vi "EOL station.vi"(0 "configuration file path":path caption="配置文件的路径", 1 "EOL station msic inf":T1) -> ()   [LabVIEW 2014]
uses:
  Ctl.xio/EOL station msic ctl.ctl
  SubVIS.xio/DataSocket/DataSocket_Tags.ctl
  Ctl.xio/part type.ctl
  <vilib>/Utility/file.llb/Read From Spreadsheet File (string).vi
  SubVIS.xio/DataSocket/Read PLC Vars/Read Bool Var.vi
  SubVIS.xio/DataSocket/Read PLC Vars/Read U32 Var.vi
  SubVIS.xio/DataSocket/Write PLC Vars/Write Bool Var in.vi
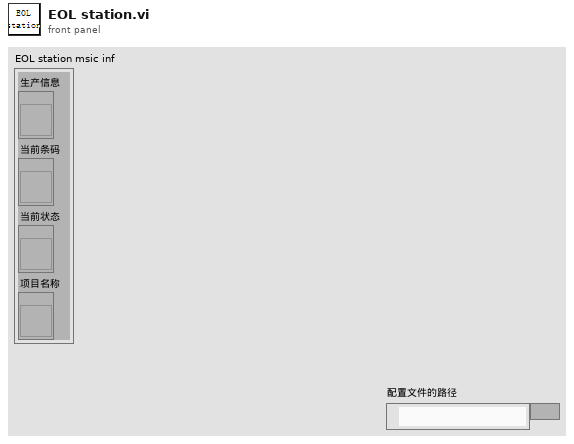
[diagram p1: front panel]
types:
  T1 = cluster{"生产信息":refnum<vi>, "当前条码":refnum<vi>, "当前状态":refnum<vi>, "项目名称":refnum<vi>}
  T2 = typedef "EOL station msic ctl.ctl" = cluster{"configuration file path":path, "DsOut":T3[], "Hopper car information":cluster{"Hopper car code":string, "Hopper car No":string, "plate No":string}, "pallet.produced number":i32, "SQL information":string, "Serial number":i32, "database path":path, "EOL station msic inf":cluster{"生产信息":refnum<vi>, "当前条码":refnum<vi>, "当前状态":refnum<vi>, "项目名称":refnum<vi>}, "part type":T4, "BarCode":string, "scanner resource name out":refnum<visa-resource-name>, "scanner coms":string, "Force value database":string[], "Force value buffer":dbl[], "SN":string, "print inf":string, "2Dcode inf":string, "Pass/Fail":bool}
  T3 = typedef "DataSocket_Tags.ctl" = cluster{"Ds ID":refnum<k13>, "Tag":string}
  T4 = typedef "part type.ctl" = cluster{"项目号":string, "物料代码":string, "零件号":string, "供应商编码":string, "产线编码":string, "客户代码":string, "颜色代码":string, "托盘上限":i32, "加热温度":string, "加热时长":string, "EOL Stations":string}
  T5 = cluster{"Hopper car code":string, "Hopper car No":string, "plate No":string}
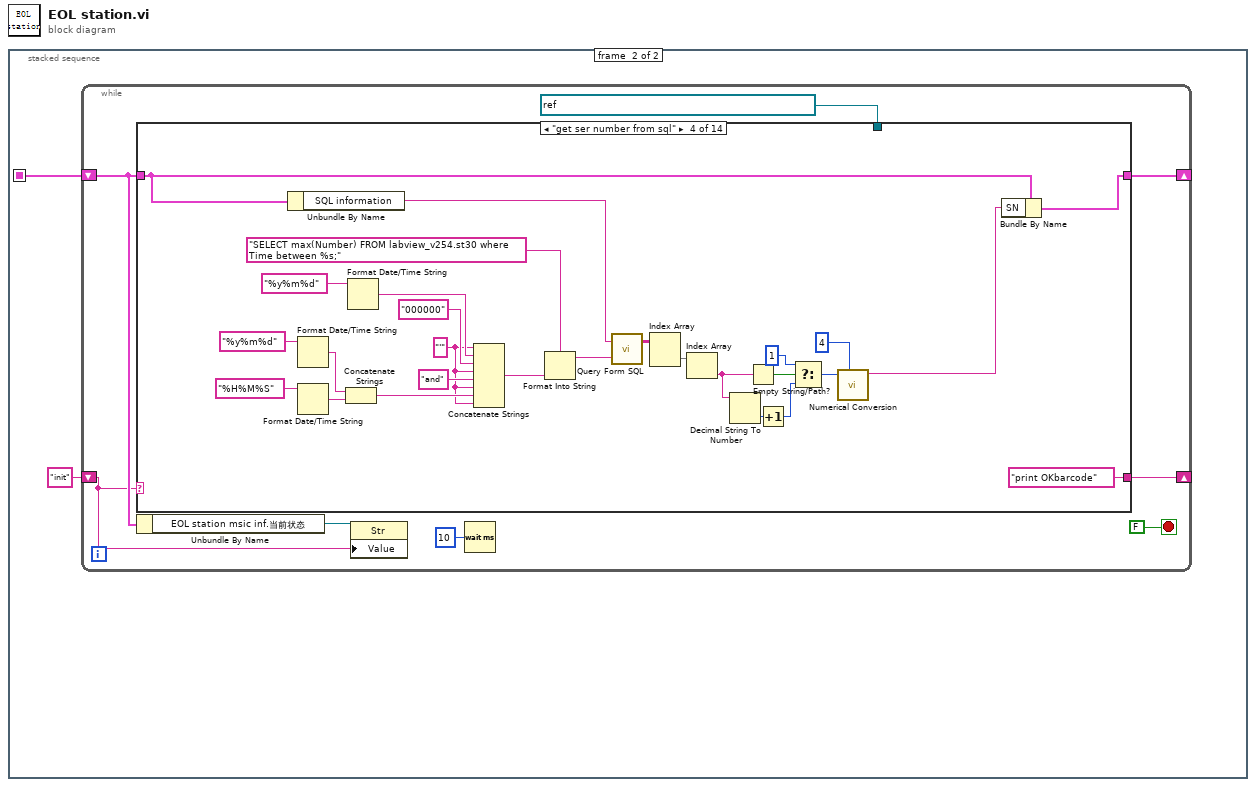
[diagram p0: block diagram]
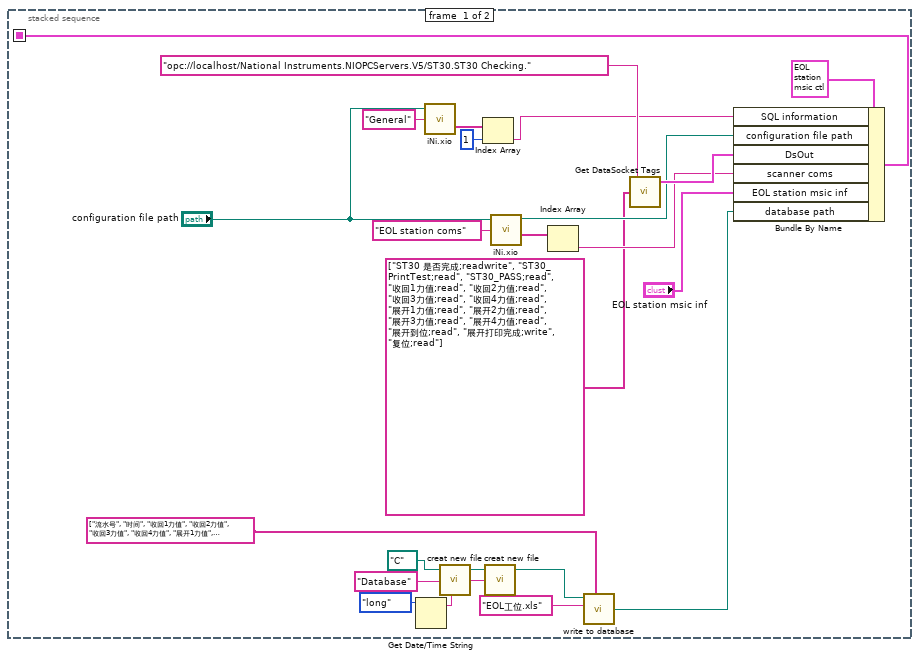
[diagram p2: hidden frame]
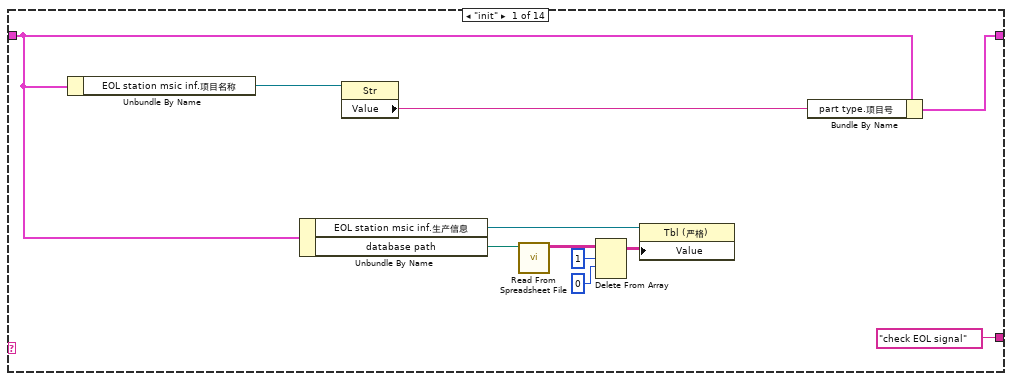
[diagram p3: hidden frame]
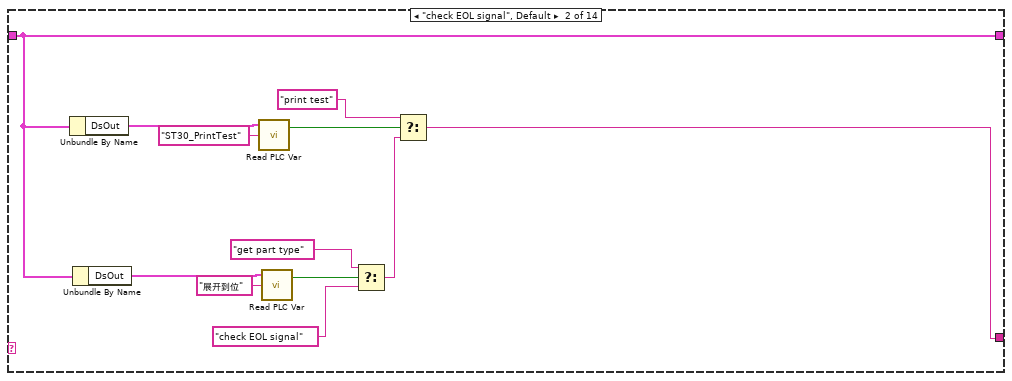
[diagram p4: hidden frame]
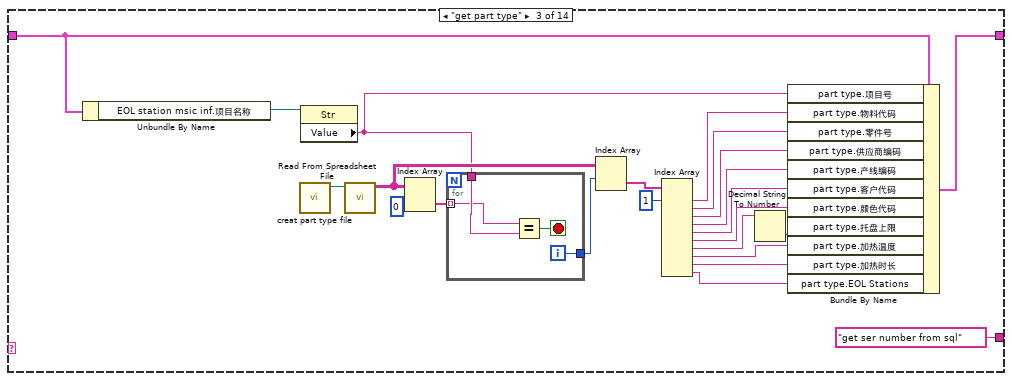
[diagram p5: hidden frame]
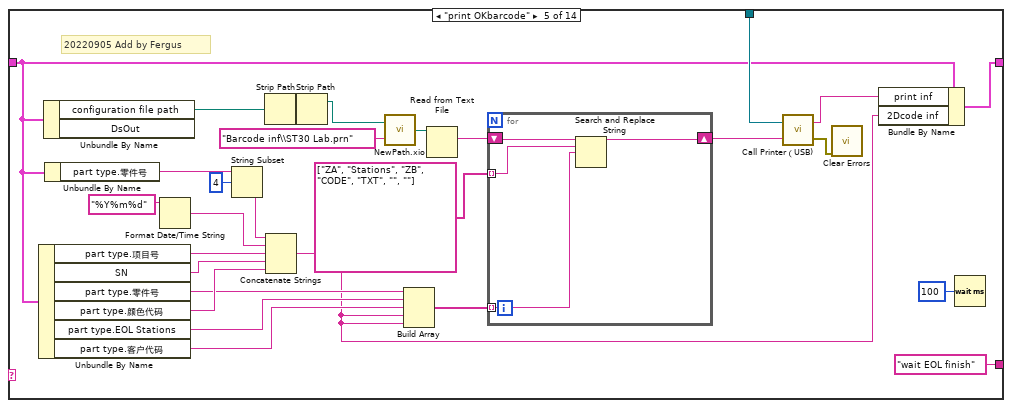
[diagram p6: hidden frame]
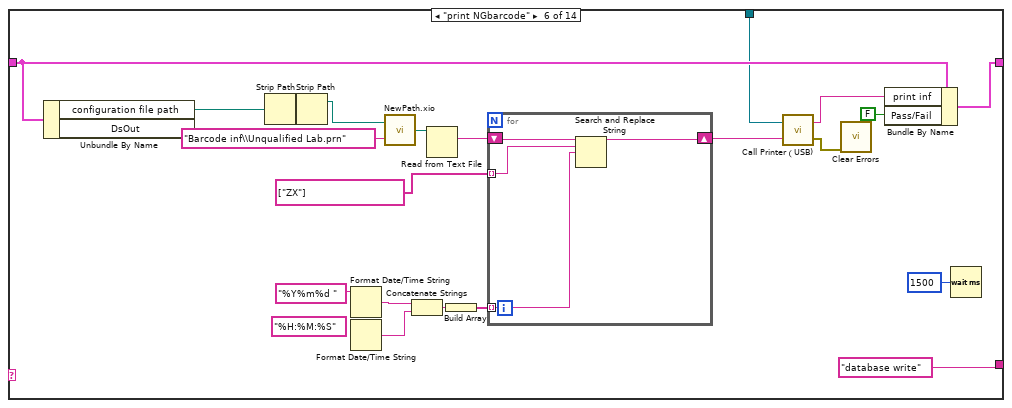
[diagram p7: hidden frame]
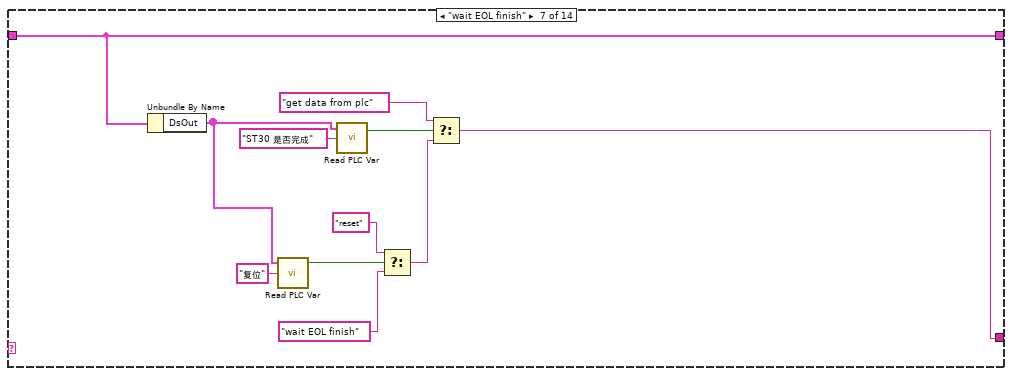
[diagram p8: hidden frame]
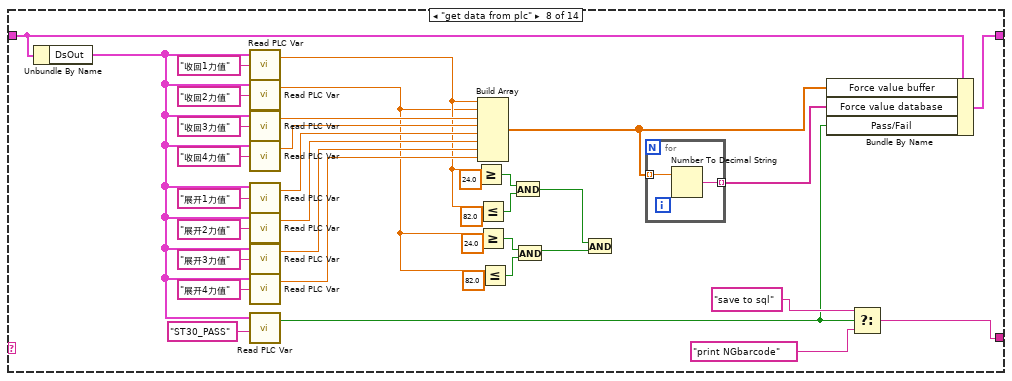
[diagram p9: hidden frame]
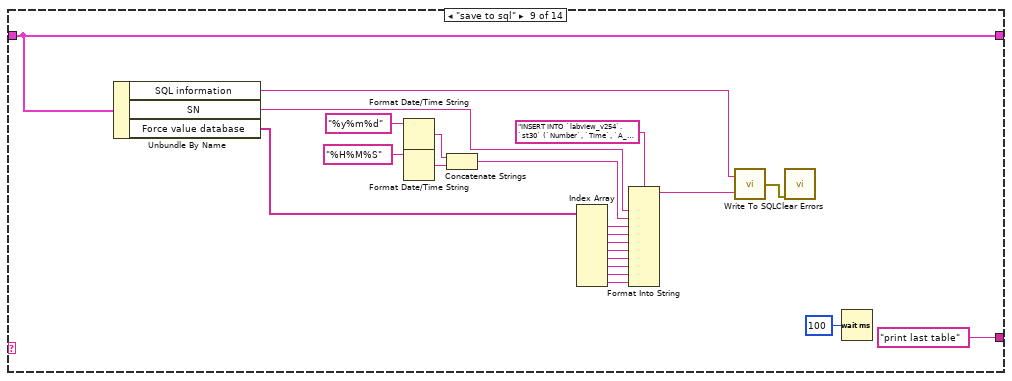
[diagram p10: hidden frame]
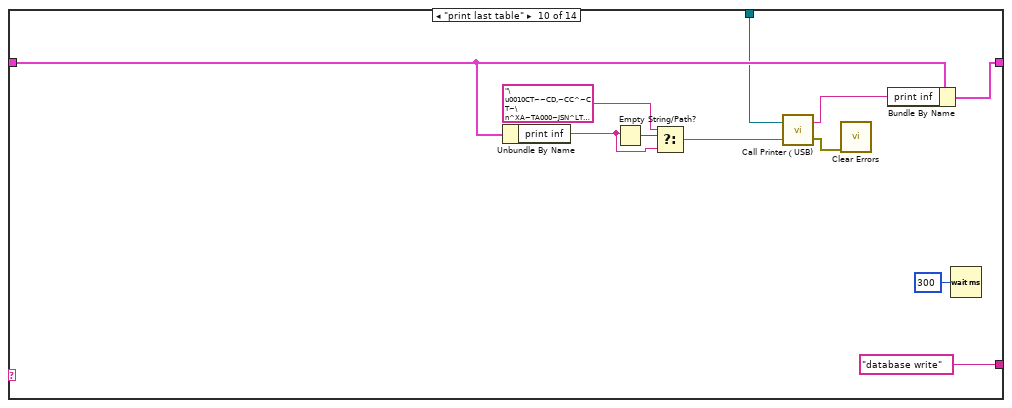
[diagram p11: hidden frame]
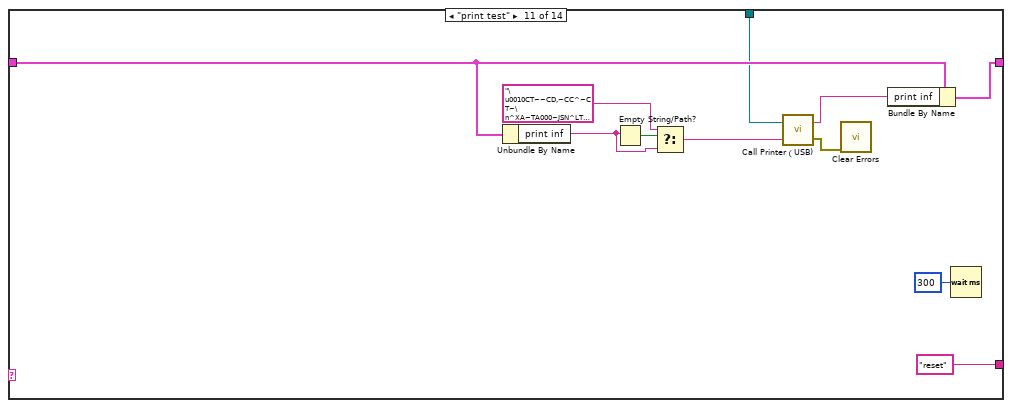
[diagram p12: hidden frame]
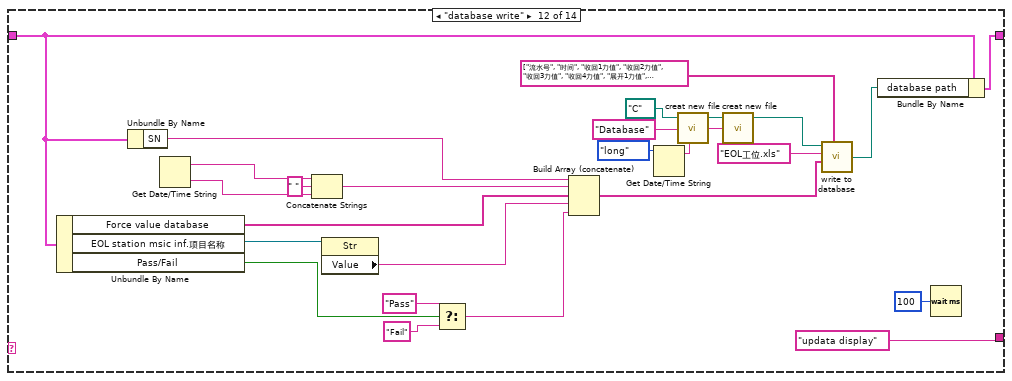
[diagram p13: hidden frame]
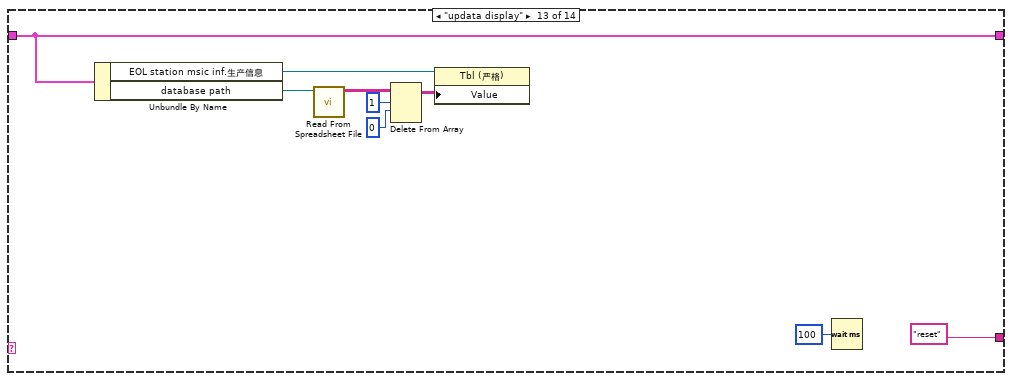
[diagram p14: hidden frame]
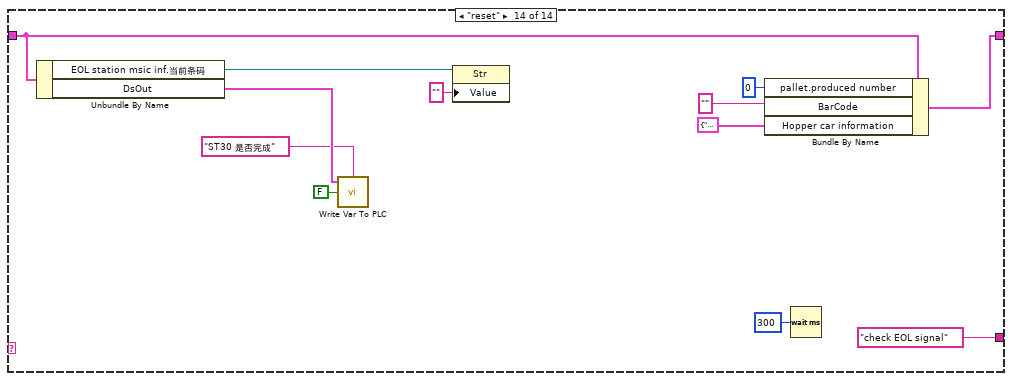
[diagram p15: hidden frame]
diagram:
  n1 = stacked-sequence {
    seq-local: [w17 _] -> [_ w25]
    frame #0 {
      n2 = Get Date/Time String(date format (0)=enum16{"short", "long", "abbreviated"}."long" ("日期格式(0)")) -> (date string=w4:string)  [unwired: 2 in, 1 out]
      n3 = call "iNi.xio.vi"("configuration file path"="configuration file path", "Sections"="General") -> ("Values"=w12:string[])  [unwired: 1 in, 4 out]
      n4 = call "creat new file.vi"("file name"="Database", "path"=path "C:/") -> ("created path"=w6:path)  [unwired: 1 in, 2 out]
      n5 = Index Array(array=w12, index=1 ("索引")) -> (element=w10:string)
      n6 = call "creat new file.vi"("file name"=w4, "path"=w6) -> ("created path"=w5:path)  [unwired: 1 in, 2 out]
      n7 = call "iNi.xio.vi"("configuration file path"="configuration file path", "Sections"="EOL station coms") -> ("configuration file path"=w23:path, "Values"=w21:string[])  [unwired: 1 in, 3 out]
      n8 = Index Array(array=w21) -> (element=w20:string)  [unwired: 1 in]
      n9 = call "write to database.vi"("Header"=string[] ["流水号", "时间", "收回1力值", "收回2力值", "收回3力值", "收回4力值", "展开1力值", "展开2力值", "展开3力值", "展开4力值", "项目号", "Pass/Fail"], "file name"="EOL工位.xls", "path"=w5) -> ("new file path (Not A Path if cancelled)"=w2:path)  [unwired: 3 in]
      n10 = call "Get DataSocket Tags.vi"("All Tags"=string[] ["ST30 是否完成;readwrite", "ST30_PrintTest;read", "ST30_PASS;read", "收回1力值;read", "收回2力值;read", "收回3力值;read", "收回4力值;read", "展开1力值;read", "展开2力值;read", "展开3力值;read", "展开4力值;read", "展开到位;read", "展开打印完成;write", "复位;read"], "URL"="opc://localhost/National Instruments.NIOPCServers.V5/ST30.ST30 Checking.") -> ("DsOut"=w24:T3[])  [unwired: 3 in]
      n11 = Bundle By Name(cluster=T2 {"configuration file path"=path "", "DsOut"=[], "Hopper car information"={"Hopper car code"="", "Hopper car No"="", "plate No"=""}, "pallet.produced number"=0, "SQL information"="", "Serial number"=0, "database path"=path "", "EOL station msic inf"={"生产信息"=refnum, "当前条码"=refnum, "当前状态"=refnum, "项目名称"=refnum}, "part type"={"项目号"="", "物料代码"="", "零件号"="", "供应商编码"="", "产线编码"="", "客户代码"="", "颜色代码"="", "托盘上限"=0, "加热温度"="", "加热时长"="", "EOL Stations"=""}, "BarCode"="", "scanner resource name out"="", "scanner coms"="", "Force value database"=[], "Force value buffer"=[], "SN"="", "print inf"="", "2Dcode inf"="", "Pass/Fail"=FALSE} ("PDF Welding msic ctl"), "SQL information"=w10, "configuration file path"=w23, "DsOut"=w24, "scanner coms"=w20, "EOL station msic inf"="EOL station msic inf", "database path"=w2) -> (w17:T2)
    }
    frame #1 {
      n12 = while {
        shift-right: [w34] -> _
        shift-left: w25 -> [w29]
        shift-right: [w33] -> _
        shift-left: "init" ("event") -> [w28]
        stop <- FALSE stop-if-true
        n13 = case shown="\"get ser number from sql\"" w28 {
          tunnel: w29 -> [w35 w50 w79 w87 w115 w155 w176 w207 w220 w246 w257 w270 w294 w303]
          tunnel: [w45 w50 w58 w90 w120 w153 w176 w206 w220 w249 w260 w283 w294 w307] -> w34
          tunnel: ["check EOL signal" w46 "get ser number from sql" ("f") "print OKbarcode" ("f") "wait EOL finish" ("f") "database write" ("f") w175 w198 "print last table" ("f") "database write" ("f") "reset" ("f") "updata display" ("f") "reset" ("f") "check EOL signal" ("f")] -> w33
          tunnel: refnum<visa-resource-name> "USB0::0x0A5F::0x0081::29J194401307::RAW" ("VISA资源名称") -> [_ _ _ _ w116 w144 _ _ _ w240 w251 _ _ _]
          frame "init" {
            n14 = Unbundle By Name(w35) -> ("EOL station msic inf.项目名称"=w44:refnum<vi>)
            n15 = Unbundle By Name(w35) -> ("EOL station msic inf.生产信息"=w41:refnum<vi>, "database path"=w40:path)
            n16 = property class="Str"(reference=w44) -> ("Value"=w43:string)  [unwired: 1 in, 2 out]
            n17 = call-poly <vilib>:"Read From Spreadsheet File.vi"("file path (dialog if empty)"=w40) -> ("all rows"=w39:string[][])  [unwired: 6 in, 4 out]
            n18 = Delete From Array(array=w39, length=1 ("长度"), index (row)=0 ("索引 (行)")) -> (array with subset deleted=w36:string[][])  [unwired: 1 in, 1 out]
            n19 = property class="Tbl (严格)"(reference=w41, "Value"=w36) -> ()  [unwired: 1 in, 2 out]
            n20 = Bundle By Name(cluster=w35, "part type.项目号"=w43) -> (w45:T2)
          }
          frame "check EOL signal", Default {
            n21 = Unbundle By Name(w50) -> ("DsOut"=w51:T3[])
            n22 = Unbundle By Name(w50) -> ("DsOut"=w57:T3[])
            n23 = call-poly "Read PLC Var.vi"("Tag IN"="ST30_PrintTest", "Ds PLCTags IN"=w51) -> ("Bool Var out"=w49:bool)  [unwired: 1 in, 1 out]
            n24 = call-poly "Read PLC Var.vi"("Tag IN"="展开到位", "Ds PLCTags IN"=w57) -> ("Bool Var out"=w55:bool)  [unwired: 1 in, 1 out]
            n25 = Select(t="get part type" ("f"), s=w55, f="check EOL signal") -> (s? t:f=w48:string)
            n26 = Select(t="print test" ("f"), s=w49, f=w48) -> (s? t:f=w46:string)
          }
          frame "get part type" {
            n27 = Unbundle By Name(w79) -> ("EOL station msic inf.项目名称"=w80:refnum<vi>)
            n28 = call "creat part type file.vi"() -> ("new file path (Not A Path if cancelled)"=w73:path)  [unwired: 11 in]
            n29 = property class="Str"(reference=w80) -> ("Value"=w72:string)  [unwired: 1 in, 2 out]
            n30 = call-poly <vilib>:"Read From Spreadsheet File.vi"("file path (dialog if empty)"=w73) -> ("all rows"=w76:string[][])  [unwired: 6 in, 4 out]
            n31 = Index Array(array=w76, index (col)=0 ("禁用的索引 (列)")) -> (element=w77:string[])  [unwired: 1 in]
            n32 = for {
              tunnel: w77 -> [w81] mode=indexing
              tunnel: [w83] -> w75
              tunnel: w72 -> [w82]
              i -> [w83]
              stop <- w84 stop-if-true
              n33 = Equal?(x=w81, y=w82) -> (x = y?=w84:bool)
            }
            n34 = Index Array(array=w76, index (row)=w75) -> (element=w74:string[])  [unwired: 1 in]
            n35 = Index Array(array=w74, index #1=1 ("索引")) -> (element #1=w69:string, element #2=w68:string, element #3=w67:string, element #4=w66:string, element #5=w64:string, element #6=w65:string, element #7=w62:string, element #8=w61:string, element #9=w60:string, element #10=w59:string)  [unwired: 9 in]
            n36 = Decimal String To Number(string=w62) -> (number=w63:i32)  [unwired: 2 in, 1 out]
            n37 = Bundle By Name(cluster=w79, "part type.项目号"=w72, "part type.物料代码"=w69, "part type.零件号"=w68, "part type.供应商编码"=w67, "part type.产线编码"=w66, "part type.客户代码"=w64, "part type.颜色代码"=w65, "part type.托盘上限"=w63, "part type.加热温度"=w61, "part type.加热时长"=w60, "part type.EOL Stations"=w59) -> (w58:T2)
          }
          frame "get ser number from sql" {
            w101 = "'" ("字符串")
            n38 = Unbundle By Name(w87) -> ("SQL information"=w86:string)
            n39 = Format Date/Time String(time format string (%c)="%y%m%d" ("时间格式字符串(%c)")) -> (date/time string=w104:string)  [unwired: 2 in]
            n40 = Format Date/Time String(time format string (%c)="%H%M%S" ("时间格式字符串(%c)")) -> (date/time string=w105:string)  [unwired: 2 in]
            n41 = Concatenate Strings(w104, w105) -> (w102:string)
            n42 = Format Date/Time String(time format string (%c)="%y%m%d" ("时间格式字符串(%c)")) -> (date/time string=w108:string)  [unwired: 2 in]
            n43 = Concatenate Strings(w101, w108, "000000" ("字符串"), w101, "and" ("字符串"), w101, w102, w101) -> (w100:string)
            n44 = Format Into String(format string="SELECT max(Number) FROM labview_v254.st30 where Time between %s;" ("SQL query"), w100) -> (resulting string=w99:string)  [unwired: 2 in, 1 out]
            n45 = call "Query Form SQL.vi"("SQL query"=w99, "SQL ID"=w86) -> ("data"=w98:string[][])  [unwired: 1 out]
            n46 = Index Array(array=w98) -> (element=w97:string[])  [unwired: 2 in]
            n47 = Index Array(array=w97) -> (element=w93:string)  [unwired: 1 in]
            n48 = Decimal String To Number(string=w93) -> (number=w92:i32)  [unwired: 2 in, 1 out]
            n49 = Empty String/Path?(string/path=w93) -> (empty?=w96:bool)
            n50 = Increment(x=w92) -> (x+1=w91:i32)
            n51 = Select(t=1, s=w96, f=w91) -> (s? t:f=w94:i32)
            n52 = call "Numerical Conversion.vi"("width"=4, "num"=w94) -> ("字符串"=w89:string)  [unwired: 9 in]
            n53 = Bundle By Name(cluster=w87, "SN"=w89) -> (w90:T2)
          }
          frame "print OKbarcode" {
            # "20220905 Add by Fergus"
            n54 = Unbundle By Name(w115) -> ("part type.项目号"=w129:string, "SN"=w123:string, "part type.零件号"=w127:string, "part type.颜色代码"=w128:string, "part type.EOL Stations"=w126:string, "part type.客户代码"=w125:string)
            n55 = Unbundle By Name(w115) -> ("configuration file path"=w138:path)  [unwired: 1 out]
            n56 = Unbundle By Name(w115) -> ("part type.零件号"=w114:string)
            n57 = Format Date/Time String(time format string (%c)="%Y%m%d" ("时间格式字符串(%c)")) -> (date/time string=w130:string)  [unwired: 2 in]
            n58 = String Subset(string=w114, offset (0)=4 ("偏移量(0)")) -> (substring=w112:string)  [unwired: 1 in]
            n59 = Strip Path(path=w138) -> (stripped path=w137:path)  [unwired: 1 out]
            n60 = Concatenate Strings(w112, w130, w129, w123, w128) -> (w119:string)
            n61 = Strip Path(path=w137) -> (stripped path=w136:path)  [unwired: 1 out]
            n62 = call "NewPath.xio.vi"("Append path"="Barcode inf\\ST30 Lab.prn", "Basic path"=w136) -> ("New path"=w134:path)
            n63 = Build Array(w127, w126, w125, w119, w119) -> (w124:string[])
            n64 = Read from Text File(file (use dialog)=w134) -> (text=w133:string)  [unwired: 3 in, 3 out]
            n65 = for {
              shift-right: [w140] -> w122
              shift-left: w133 -> [w143]
              tunnel: string[] ["ZA", "Stations", "ZB", "CODE", "TXT", "", ""] -> [w142] mode=indexing
              tunnel: w124 -> [w141] mode=indexing
              n66 = Search and Replace String(input string=w143, search string=w142, replace string=w141) -> (result string=w140:string)  [unwired: 5 in, 3 out]
            }
            n67 = call "Call Printer（USB).vi"("写入缓冲区"=w122, "VISA资源名称"=w116) -> ("error out"=w118:errorcluster, "Last P"=w121:string)
            n68 = call <vilib>:"Clear Errors.vi"("error in (no error)"=w118) -> ()  [unwired: 5 in, 2 out]
            n69 = Bundle By Name(cluster=w115, "print inf"=w121, "2Dcode inf"=w119) -> (w120:T2)
            n70 = Wait (ms)(milliseconds to wait=u32 100 ("等待时间（毫秒）")) -> ()  [unwired: 1 out]
          }
          frame "print NGbarcode" {
            (unwired) "%H:%M:%S" ("时间格式字符串(%c)")
            n71 = Unbundle By Name(w155) -> ("configuration file path"=w164:path)  [unwired: 1 out]
            n72 = Strip Path(path=w164) -> (stripped path=w163:path)  [unwired: 1 out]
            n73 = Strip Path(path=w163) -> (stripped path=w162:path)  [unwired: 1 out]
            n74 = Format Date/Time String(time format string (%c)="%Y%m%d " ("时间格式字符串(%c)")) -> (date/time string=w151:string)  [unwired: 2 in]
            n75 = Format Date/Time String() -> (date/time string=w150:string)  [unwired: 3 in]
            n76 = call "NewPath.xio.vi"("Append path"="Barcode inf\\Unqualified Lab.prn", "Basic path"=w162) -> ("New path"=w160:path)
            n77 = Concatenate Strings(w151, w150) -> (w149:string)
            n78 = Read from Text File(file (use dialog)=w160) -> (text=w159:string)  [unwired: 3 in, 3 out]
            n79 = Build Array(w149) -> (w157:string[])
            n80 = for {
              shift-right: [w165] -> w156
              shift-left: w159 -> [w168]
              tunnel: string[] ["ZX"] -> [w167] mode=indexing
              tunnel: w157 -> [w166] mode=indexing
              n81 = Search and Replace String(input string=w168, search string=w167, replace string=w166) -> (result string=w165:string)  [unwired: 5 in, 3 out]
            }
            n82 = call "Call Printer（USB).vi"("写入缓冲区"=w156, "VISA资源名称"=w144) -> ("error out"=w148:errorcluster, "Last P"=w154:string)
            n83 = call <vilib>:"Clear Errors.vi"("error in (no error)"=w148) -> ()  [unwired: 5 in, 2 out]
            n84 = Bundle By Name(cluster=w155, "print inf"=w154, "Pass/Fail"=FALSE) -> (w153:T2)
            n85 = Wait (ms)(milliseconds to wait=u32 1500 ("等待时间（毫秒）")) -> ()  [unwired: 1 out]
          }
          frame "wait EOL finish" {
            n86 = Unbundle By Name(w176) -> ("DsOut"=w173:T3[])
            n87 = call-poly "Read PLC Var.vi"("Tag IN"="复位", "Ds PLCTags IN"=w173) -> ("Bool Var out"=w172:bool)  [unwired: 1 in, 1 out]
            n88 = call-poly "Read PLC Var.vi"("Tag IN"="ST30 是否完成", "Ds PLCTags IN"=w173) -> ("Bool Var out"=w178:bool)  [unwired: 1 in, 1 out]
            n89 = Select(t="reset" ("f"), s=w172, f="wait EOL finish") -> (s? t:f=w169:string)
            n90 = Select(t="get data from plc" ("f"), s=w178, f=w169) -> (s? t:f=w175:string)
          }
          frame "get data from plc" {
            n91 = Unbundle By Name(w207) -> ("DsOut"=w183:T3[])
            n92 = call-poly "Read PLC Var.vi"("Tag IN"="收回1力值", "Ds PLCTags IN"=w183) -> ("U32 Var out"=w194:dbl)  [unwired: 1 in, 1 out]
            n93 = call-poly "Read PLC Var.vi"("Tag IN"="收回2力值", "Ds PLCTags IN"=w183) -> ("U32 Var out"=w186:dbl)  [unwired: 1 in, 1 out]
            n94 = call-poly "Read PLC Var.vi"("Tag IN"="收回3力值", "Ds PLCTags IN"=w183) -> ("U32 Var out"=w205:dbl)  [unwired: 1 in, 1 out]
            n95 = call-poly "Read PLC Var.vi"("Tag IN"="收回4力值", "Ds PLCTags IN"=w183) -> ("U32 Var out"=w204:dbl)  [unwired: 1 in, 1 out]
            n96 = call-poly "Read PLC Var.vi"("Tag IN"="展开1力值", "Ds PLCTags IN"=w183) -> ("U32 Var out"=w200:dbl)  [unwired: 1 in, 1 out]
            n97 = call-poly "Read PLC Var.vi"("Tag IN"="展开2力值", "Ds PLCTags IN"=w183) -> ("U32 Var out"=w203:dbl)  [unwired: 1 in, 1 out]
            n98 = call-poly "Read PLC Var.vi"("Tag IN"="展开3力值", "Ds PLCTags IN"=w183) -> ("U32 Var out"=w202:dbl)  [unwired: 1 in, 1 out]
            n99 = call-poly "Read PLC Var.vi"("Tag IN"="展开4力值", "Ds PLCTags IN"=w183) -> ("U32 Var out"=w201:dbl)  [unwired: 1 in, 1 out]
            n100 = call-poly "Read PLC Var.vi"("Tag IN"="ST30_PASS", "Ds PLCTags IN"=w183) -> ("Bool Var out"=w180:bool)  [unwired: 1 in, 1 out]
            n101 = Greater Or Equal?(x=w194, y=24.0) -> (x >= y?=w191:bool)
            n102 = Build Array(w194, w186, w205, w204, w200, w203, w202, w201) -> (w197:dbl[])
            n103 = Less Or Equal?(x=w194, y=82.0) -> (x <= y?=w192:bool)
            n104 = Greater Or Equal?(x=w186, y=24.0) -> (x >= y?=w190:bool)
            n105 = Less Or Equal?(x=w186, y=82.0) -> (x <= y?=w189:bool)
            n106 = And(x=w191, y=w192) -> (x .and. y?=w184:bool)
            n107 = And(x=w190, y=w189) -> (x .and. y?=w185:bool)
            n108 = And(x=w184, y=w185) -> ()  [unwired: 1 out]
            n109 = for {
              tunnel: w197 -> [w217] mode=indexing
              tunnel: [w216] -> w196 mode=indexing
              n110 = Number To Decimal String(number=w217) -> (decimal integer string=w216:string)  [unwired: 1 in]
            }
            n111 = Bundle By Name(cluster=w207, "Force value buffer"=w197, "Force value database"=w196, "Pass/Fail"=w180) -> (w206:T2)
            n112 = Select(t="save to sql" ("f"), s=w180, f="print NGbarcode") -> (s? t:f=w198:string)
          }
          frame "save to sql" {
            n113 = Unbundle By Name(w220) -> ("SQL information"=w222:string, "SN"=w234:string, "Force value database"=w233:string[])
            n114 = Format Date/Time String(time format string (%c)="%y%m%d" ("时间格式字符串(%c)")) -> (date/time string=w237:string)  [unwired: 2 in]
            n115 = Format Date/Time String(time format string (%c)="%H%M%S" ("时间格式字符串(%c)")) -> (date/time string=w238:string)  [unwired: 2 in]
            n116 = Concatenate Strings(w237, w238) -> (w235:string)
            n117 = Index Array(array=w233) -> (element #1=w232:string, element #2=w231:string, element #3=w230:string, element #4=w229:string, element #5=w228:string, element #6=w227:string, element #7=w226:string, element #8=w225:string)  [unwired: 8 in]
            n118 = Format Into String(format string="INSERT INTO `labview_v254`.`st30` (`Number`, `Time`, `A_Data1`, `A_Data2`, `A_Data3`, `A_Data4`, `B_Data1`, `B_Data2`, `B_Data3`, `B_Data4`) VALUES ('%s', '%s', '%s', '%s', '%s', '%s', '%s', '%s', '%s', '%s');" ("初始字符串"), w234, w235, w232, w231, w230, w229, w228, w227, w226, w225) -> (resulting string=w223:string)  [unwired: 2 in, 1 out]
            n119 = call "Write To SQL.vi"("SQL query"=w223, "connection information"=w222) -> ("error out"=w221:errorcluster)
            n120 = call <vilib>:"Clear Errors.vi"("error in (no error)"=w221) -> ()  [unwired: 5 in, 2 out]
            n121 = Wait (ms)(milliseconds to wait=u32 100 ("等待时间（毫秒）")) -> ()  [unwired: 1 out]
          }
          frame "print last table" {
            n122 = Unbundle By Name(w246) -> ("print inf"=w243:string)
            n123 = Empty String/Path?(string/path=w243) -> (empty?=w245:bool)
            n124 = Select(t="\u0010CT~~CD,~CC^~CT~\n^XA~TA000~JSN^LT0^MNW^MTT^PON^PMN^LH0,0^JMA^PR5,5~SD15^JUS^LRN^CI0^XZ\n~DG000.GRF,00768,024,\n,::I07,I0780I0J8H0LA80H0E0I0380E,I0380I0IFE007FJF8001E0I0181C,02ABAA800EAAE002H2E228003F0I038380I0F0,07FIFC00C0060I01C0J0H3J0101FF80070,H0K8H0E00E0I01C0J0FBC0H0383AF800F0,H0701C0H0C0060I01C0J0E1C0017D7870H070,H0781E0H0E00E0I0380I03E0F003FHF870H0F0,H0301C0H0C0060I0780I0380780031DC70H070,H03C380H0IFE0I0F9C0H0F803E0078CEE0H0F0,J030P01FDE001E0H0FC07C07C0H070,0FJFE0N03B8F007BFHF3C0FE0380H0E0,07FIFE0N071870071J1H07F07E0H070,0E0K0HFEFFE00FB83C020L0HFBEFE00E0,070K0HFC7FE01C1C1E0M01F9F01E0060,0E0K0E0EE0E038380F003BHB803B9E00E0060,060K0C0C60607018070075H5C01907FF8,0E0K0E0EE0E0E0380200E001C03B838B8,0E0K0C0C6060H01C0I07001C01187018,0E0K0E0EE0E0H0380I0E001C00383038,1C0K0C0C6060H0180I07001C001070180070,1E0K0HFEFFE0H0380I0FAABC0038783800F0,1C0K0HFC7FE0H01C0I07FHFC00187D7800F0,380K0E0EE060H0380I0E003C00383AB8,30L040440J0180I07001C00107018,X080I0A0H0800282828,,::^XA\n^MMT\n^PW719\n^LL0096\n^LS0\n^FT166,88^A0N,20,21^FH\\^FDZX^FS\n^FT416,64^XG000.GRF,1,1^FS\n^FT78,88^A0N,20,21^FH\\^FDSerial nr:^FS\n^FT142,44^A0N,28,28^FH\\^FDNok^FS\n^PQ1,0,1,Y^XZ\n^XA^ID000.GRF^FS^XZ", s=w245, f=w243) -> (s? t:f=w242:string)
            n125 = call "Call Printer（USB).vi"("写入缓冲区"=w242, "VISA资源名称"=w240) -> ("error out"=w248:errorcluster, "Last P"=w250:string)
            n126 = call <vilib>:"Clear Errors.vi"("error in (no error)"=w248) -> ()  [unwired: 5 in, 2 out]
            n127 = Bundle By Name(cluster=w246, "print inf"=w250) -> (w249:T2)
            n128 = Wait (ms)(milliseconds to wait=u32 300 ("等待时间（毫秒）")) -> ()  [unwired: 1 out]
          }
          frame "print test" {
            n129 = Unbundle By Name(w257) -> ("print inf"=w254:string)
            n130 = Empty String/Path?(string/path=w254) -> (empty?=w256:bool)
            n131 = Select(t="\u0010CT~~CD,~CC^~CT~\n^XA~TA000~JSN^LT0^MNW^MTT^PON^PMN^LH0,0^JMA^PR5,5~SD15^JUS^LRN^CI0^XZ\n~DG000.GRF,00768,024,\n,::I07,I0780I0J8H0LA80H0E0I0380E,I0380I0IFE007FJF8001E0I0181C,02ABAA800EAAE002H2E228003F0I038380I0F0,07FIFC00C0060I01C0J0H3J0101FF80070,H0K8H0E00E0I01C0J0FBC0H0383AF800F0,H0701C0H0C0060I01C0J0E1C0017D7870H070,H0781E0H0E00E0I0380I03E0F003FHF870H0F0,H0301C0H0C0060I0780I0380780031DC70H070,H03C380H0IFE0I0F9C0H0F803E0078CEE0H0F0,J030P01FDE001E0H0FC07C07C0H070,0FJFE0N03B8F007BFHF3C0FE0380H0E0,07FIFE0N071870071J1H07F07E0H070,0E0K0HFEFFE00FB83C020L0HFBEFE00E0,070K0HFC7FE01C1C1E0M01F9F01E0060,0E0K0E0EE0E038380F003BHB803B9E00E0060,060K0C0C60607018070075H5C01907FF8,0E0K0E0EE0E0E0380200E001C03B838B8,0E0K0C0C6060H01C0I07001C01187018,0E0K0E0EE0E0H0380I0E001C00383038,1C0K0C0C6060H0180I07001C001070180070,1E0K0HFEFFE0H0380I0FAABC0038783800F0,1C0K0HFC7FE0H01C0I07FHFC00187D7800F0,380K0E0EE060H0380I0E003C00383AB8,30L040440J0180I07001C00107018,X080I0A0H0800282828,,::^XA\n^MMT\n^PW719\n^LL0096\n^LS0\n^FT166,88^A0N,20,21^FH\\^FDZX^FS\n^FT416,64^XG000.GRF,1,1^FS\n^FT78,88^A0N,20,21^FH\\^FDSerial nr:^FS\n^FT142,44^A0N,28,28^FH\\^FDNok^FS\n^PQ1,0,1,Y^XZ\n^XA^ID000.GRF^FS^XZ", s=w256, f=w254) -> (s? t:f=w253:string)
            n132 = call "Call Printer（USB).vi"("写入缓冲区"=w253, "VISA资源名称"=w251) -> ("error out"=w259:errorcluster, "Last P"=w261:string)
            n133 = call <vilib>:"Clear Errors.vi"("error in (no error)"=w259) -> ()  [unwired: 5 in, 2 out]
            n134 = Bundle By Name(cluster=w257, "print inf"=w261) -> (w260:T2)
            n135 = Wait (ms)(milliseconds to wait=u32 300 ("等待时间（毫秒）")) -> ()  [unwired: 1 out]
          }
          frame "database write" {
            n136 = Unbundle By Name(w270) -> ("Force value database"=w271:string[], "EOL station msic inf.项目名称"=w269:refnum<vi>, "Pass/Fail"=w265:bool)
            n137 = Unbundle By Name(w270) -> ("SN"=w278:string)
            n138 = Get Date/Time String() -> (date string=w274:string, time string=w273:string)  [unwired: 3 in]
            n139 = Concatenate Strings(w274, " " ("字符串"), w273) -> (w277:string)
            n140 = property class="Str"(reference=w269) -> ("Value"=w268:string)  [unwired: 1 in, 2 out]
            n141 = Select(t="Pass", s=w265, f="Fail") -> (s? t:f=w262:string)
            n142 = Build Array (concatenate)(w278, w277, w271, w268, w262) -> (w276:string[])
            n143 = Get Date/Time String(date format (0)=enum16{"short", "long", "abbreviated"}."long" ("日期格式(0)")) -> (date string=w280:string)  [unwired: 2 in, 1 out]
            n144 = call "creat new file.vi"("file name"="Database", "path"=path "C:/") -> ("created path"=w282:path)  [unwired: 1 in, 2 out]
            n145 = call "creat new file.vi"("file name"=w280, "path"=w282) -> ("created path"=w281:path)  [unwired: 1 in, 2 out]
            n146 = call "write to database.vi"("Header"=string[] ["流水号", "时间", "收回1力值", "收回2力值", "收回3力值", "收回4力值", "展开1力值", "展开2力值", "展开3力值", "展开4力值", "项目号", "Pass/Fail"], "data in"=w276, "file name"="EOL工位.xls", "path"=w281) -> ("new file path (Not A Path if cancelled)"=w284:path)  [unwired: 2 in]
            n147 = Bundle By Name(cluster=w270, "database path"=w284) -> (w283:T2)
            n148 = Wait (ms)(milliseconds to wait=u32 100 ("等待时间（毫秒）")) -> ()  [unwired: 1 out]
          }
          frame "updata display" {
            n149 = Unbundle By Name(w294) -> ("EOL station msic inf.生产信息"=w296:refnum<vi>, "database path"=w295:path)
            n150 = call-poly <vilib>:"Read From Spreadsheet File.vi"("file path (dialog if empty)"=w295) -> ("all rows"=w293:string[][])  [unwired: 6 in, 4 out]
            n151 = Delete From Array(array=w293, length=1 ("长度"), index (row)=0 ("索引 (行)")) -> (array with subset deleted=w290:string[][])  [unwired: 1 in, 1 out]
            n152 = property class="Tbl (严格)"(reference=w296, "Value"=w290) -> ()  [unwired: 1 in, 2 out]
            n153 = Wait (ms)(milliseconds to wait=u32 100 ("等待时间（毫秒）")) -> ()  [unwired: 1 out]
          }
          frame "reset" {
            n154 = Unbundle By Name(w303) -> ("EOL station msic inf.当前条码"=w302:refnum<vi>, "DsOut"=w299:T3[])
            n155 = call-poly "Write Var To PLC.vi"("Tag IN"="ST30 是否完成", "Bool Var in"=FALSE, "Ds PLCTags IN"=w299) -> ()  [unwired: 1 in, 2 out]
            n156 = property class="Str"(reference=w302, "Value"="" ("值")) -> ()  [unwired: 1 in, 2 out]
            n157 = Bundle By Name(cluster=w303, "pallet.produced number"=0, "BarCode"="", "Hopper car information"=T5 {"Hopper car code"="", "Hopper car No"="", "plate No"=""}) -> (w307:T2)
            n158 = Wait (ms)(milliseconds to wait=u32 300 ("等待时间（毫秒）")) -> ()  [unwired: 1 out]
          }
        }
        n159 = Unbundle By Name(w29) -> ("EOL station msic inf.当前状态"=w30:refnum<vi>)
        n160 = property class="Str"(reference=w30, "Value"=w28) -> ()  [unwired: 1 in, 2 out]
        n161 = Wait (ms)(milliseconds to wait=u32 10 ("等待时间（毫秒）")) -> ()  [unwired: 1 out]
      }
    }
  }
